vi "PH_AxisGUI_BaseClass.constructor.vi"(0 "name":string, 2 "data in":string, 5 "error in(no error)":errorcluster) -> (14 "i ref out":refnum<vi>, 16 "data out":string, 19 "error out":errorcluster)   [LabVIEW 2014, in "PH_AxisGUI_BaseClass.lvlib"]
doc: "This class is forseen to control motion Axes.\n\nThis class is part of the PHELIX device layer.\n\nauthor: Stefan Götte, GSI\n\nLicense Agreement for this software:\n\nCopyright (C)\nGesellschaft für Schwerionenforschung, GSI\nPlanckstr. 1\n64291 Darmstadt\nGermany\n\nContact: D.Beck@gsi.de \n\nThis program is free software; you can redistribute it and/or modify it under the terms of the \nGNU General Public License as published by the Free Software Foundation; either version 2 of \nthe license, or (at your option) any later version.\n\nThis program is distributed in the hope that it will be useful, but WITHOUT ANY WARRANTY; \nwithout even the implied warranty of MERCHANTABILITY or FITNESS FOR A PARTICULAR PURPOSE. See the GNU General License for more details (http://www.gnu.org).\n\nGesellschaft für Schwerionenforschung, GSI\nPlanckstr. 1, 64291 Darmstadt, Germany\nFor all questions and ideas contact: M.Richter@gsi.de, H.Brand@gsi.de or D.Beck@gsi.de.\nLast update: 16-JUN-2004"
uses:
  PH_AxisGUI_BaseClass.lvlib
  CS_Core/CSSystem/CSSystemLib/CSSystemLib.lvlib
  PH_Class/PH_Class.lvlib
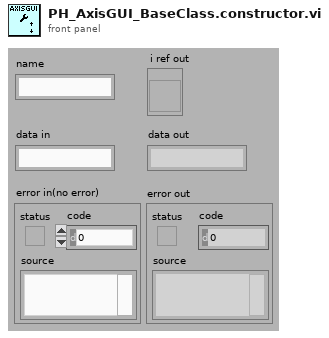
[diagram p1: front panel]
types:
  T1 = enum16{"SetAttribute", "GetAttribute", "CreateAttribute", "DestroyAttribute", "DestroyAllAtributes"}
  T2 = typedef "PH_AxisGUI_BaseClass.lvlib/PH_AxisGUI_BaseClass.i attribute.ctl" = cluster{"Axes":T3[]}
  T3 = typedef "PH_AxisGUI_BaseClass.lvlib/PH_AxisGUI_BaseClass.Axis Attributes.ctl" = cluster{"Axis GUI Refs":T4, "Address":T5, "Name":string, "Label \"Back\"":string, "Labell \"Forth\"":string, "Moving?":bool}
  T4 = typedef "PH_AxisGUI_BaseClass.lvlib/PH_AxisGUI_BaseClass.Axis GUI Refs.ctl" = cluster{"Back":refnum<vi>, "Forth":refnum<vi>, "Status":refnum<vi>, "Target":refnum<vi>, "Address":refnum<vi>, "Status Bar":refnum<vi>, "Settings":refnum<vi>, "Activity":refnum<vi>, "Clear Error":refnum<vi>}
  T5 = typedef "PH_Stepmotor_BaseClass.lvlib/PH_Stepmotor_BaseClass.Axis Address.ctl" = cluster{"Instance":string, "Motor Nr":i32}
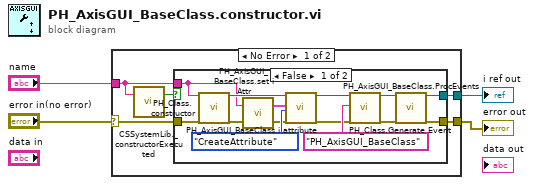
[diagram p0: block diagram]
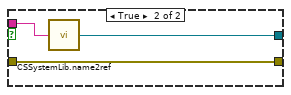
[diagram p2: hidden frame]
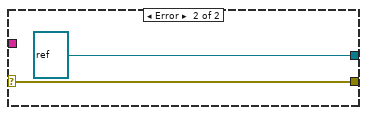
[diagram p3: hidden frame]
diagram:
  n1 = case shown="No Error" "error in(no error)" {
    selector: "error in(no error)" -> [w9 w28]
    tunnel: [w7 w28] -> w4
    tunnel: [w8 refnum<vi> refnum ("i ref out")] -> w3
    tunnel: "name" -> [w6 _]
    frame No Error {
      n2 = call "CSSystemLib._constructorExecuted.vi"("name"=w6) -> ("constructor executed?"=w5:bool)  [unwired: 18 in]
      n3 = case shown="False" w5 {
        tunnel: w9 -> [w12 w26]
        tunnel: [w21 w24] -> w8
        tunnel: [w20 w26] -> w7
        tunnel: w6 -> [w14 w25]
        frame False {
          n4 = call "PH_Class.constructor.vi"("name"=w14, "error in"=w12) -> ("i ref out"=w22:refnum<vi>, "error out"=w11:errorcluster)  [unwired: 15 in, 1 out]
          n5 = call "PH_AxisGUI_BaseClass.set i Attr.vi"("error in (no error)"=w11, "Instance Name"=w14) -> ("error out"=w10:errorcluster, "i Attributes"=w13:T2)
          n6 = call "PH_AxisGUI_BaseClass.i attribute.vi"("VI Refnum"=w22, "CLASS.i attribute"=w13, "Action"=T1."CreateAttribute", "error in (no error)"=w10) -> ("VI Refnum out"=w18:refnum<vi>, "error out"=w16:errorcluster)  [unwired: 13 in, 1 out]
          n7 = call "PH_Class.Generate Event.vi"("i ref in"=w18, "Class"="PH_AxisGUI_BaseClass", "error in (no error)"=w16) -> ("i ref out"=w17:refnum<vi>, "error out"=w15:errorcluster)  [unwired: 15 in]
          n8 = call "PH_AxisGUI_BaseClass.ProcEvents.vi"("i ref in"=w17, "error in"=w15) -> ("i ref out"=w21:refnum<vi>, "error out"=w20:errorcluster)  [unwired: 16 in]
        }
        frame True {
          n9 = call "CSSystemLib.name2ref.vi"("name"=w25) -> ("obj refnum"=w24:refnum<vi>)
        }
      }
    }
    frame Error {
    }
  }
  "i ref out" <- w3
  "error out" <- w4
